vi "Timer.vi"(1 "Start Timer":bool) -> (0 "Time elapsed":u64)   [LabVIEW 2014]
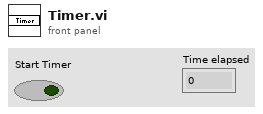
[diagram p1: front panel]
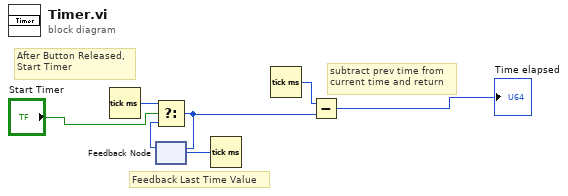
[diagram p0: block diagram]
diagram:
  # "After Button Released,\nStart Timer"
  # "Feedback Last Time Value"
  # "subtract prev time from\ncurrent time and return"
  n1 = Tick Count (ms)() -> (millisecond timer value=w4:u32)
  n2 = Tick Count (ms)() -> (millisecond timer value=w6:u32)
  n3 = feedback #1(w6) -> (w5:u32)
  n4 = Select(t=w4, s="Start Timer", f=w5) -> (s? t:f=w2:u32)
  n5 = feedback-in #1(w2) -> ()
  n6 = Tick Count (ms)() -> (millisecond timer value=w3:u32)
  n7 = Subtract(x=w3, y=w2) -> (x-y=→"Time elapsed":u32)
